vi "MAV_CMD_DO_SET_RELAY.vi"(9 "Set Relay (T:ON)":bool, 10 "Relay  Number":sgl, 11 "Target System and Target Component":u8=1) -> (3 "MAVLink Message":u8[](array[numeric]))   [LabVIEW 2014]
panel:
  out "Payload Size":i32
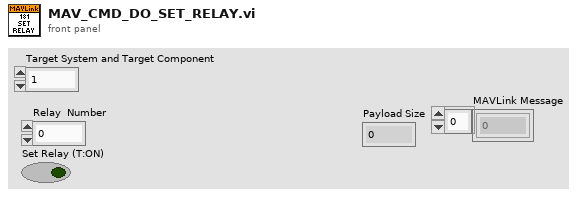
[diagram p1: front panel]
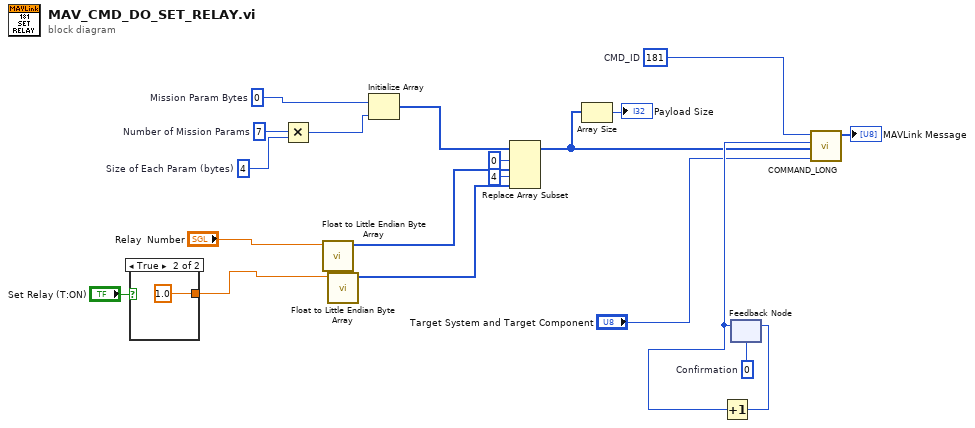
[diagram p0: block diagram]
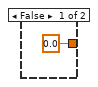
[diagram p2: hidden frame]
diagram:
  w13 = u8 0  # Confirmation
  w18 = 4  # Size of Each Param (bytes)
  w19 = 7  # Number of Mission Params
  w20 = u8 0  # Mission Param Bytes
  w9 = u16 181  # CMD_ID
  n1 = case shown="True" "Set Relay (T:ON)" {
    tunnel: [sgl 0.0 sgl 1.0] -> w1
    frame False {
    }
    frame True {
    }
  }
  n2 = Multiply(x=w19, y=w18) -> (x*y=w17:i32)
  n3 = call "Float to Little Endian Byte Array.vi"("Float In"="Relay  Number") -> ("LE Byte Array"=w10:u8[])  [unwired: 10 in]
  n4 = call "Float to Little Endian Byte Array.vi"("Float In"=w1) -> ("LE Byte Array"=w4:u8[])  [unwired: 10 in]
  n5 = Initialize Array(w20, w17) -> (w16:u8[])
  n6 = Replace Array Subset(array=w16, new element #1=w10, index #1=0 ("index"), new element #2=w4, index #2=4 ("index")) -> (w7:u8[])
  n7 = Array Size(array=w7) -> (size(s)=→"Payload Size":i32)
  n8 = feedback #1(w13) -> (w8:u8)
  n9 = Increment(x=w8) -> (x+1=w12:u8)
  n10 = feedback-in #1(w12) -> ()
  n11 = call "COMMAND_LONG.vi"("Target System and Target Component"="Target System and Target Component", "Mission Params"=w7, "Confirmation"=w8, "Command ID"=w9) -> ("MAVLink Message"=→"MAVLink Message":u8[])  [unwired: 7 in]
